vi "Flow_2_Buffer_Dbl_VIG.vi"(7 "Operation":enum16{"get data", "set data", "initialize"}(ring)=enum."set data", 8 "error in":errorcluster, 11 "Freq":dbl) -> (0 "error out":errorcluster, 3 "Raw Flow Freq":dbl)   [LabVIEW 2018]
uses:
  <vilib>/Analysis/baseanly.llb/Mean (DBL).vi
  <vilib>/measure/macond.llb/FIR Filter for 1 Chan.vi
  Common/Globals/Flow Global.vi
  <vilib>/gmath/NI_Gmath.lvlib
  <vilib>/measure/NI_MAPro.lvlib
  <vilib>/Analysis/NI_AALBase.lvlib
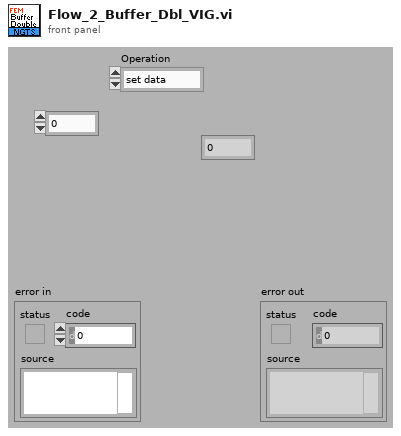
[diagram p1: front panel]
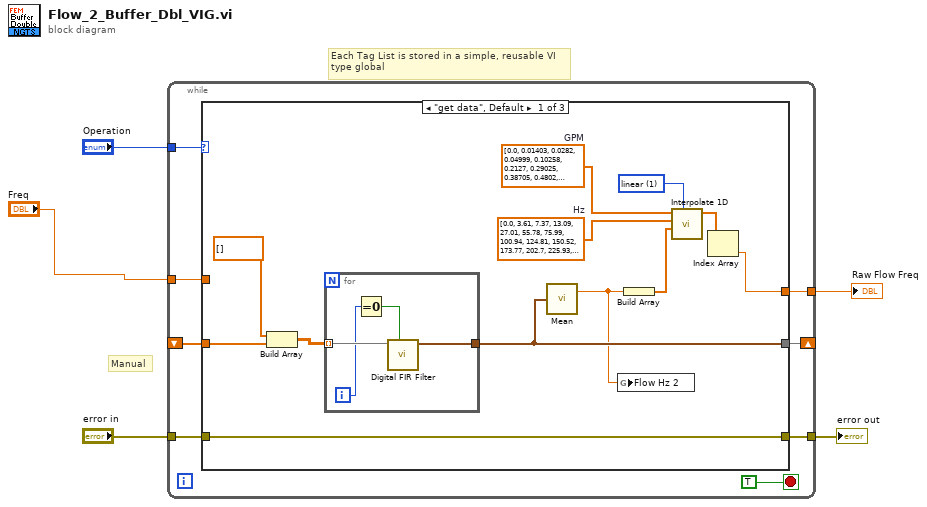
[diagram p0: block diagram]
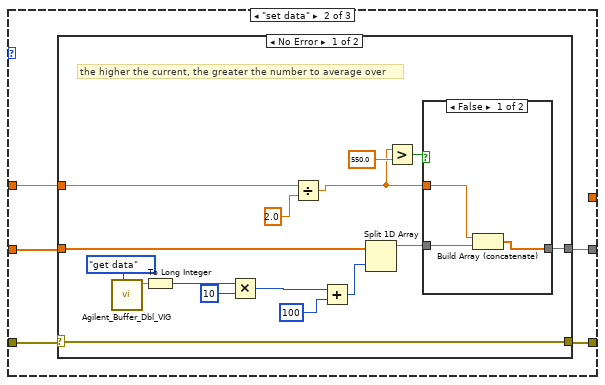
[diagram p2: hidden frame]
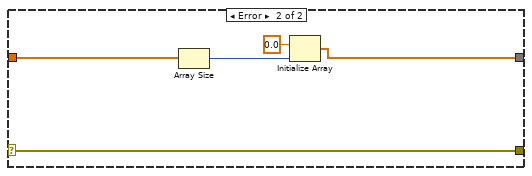
[diagram p4: hidden frame]
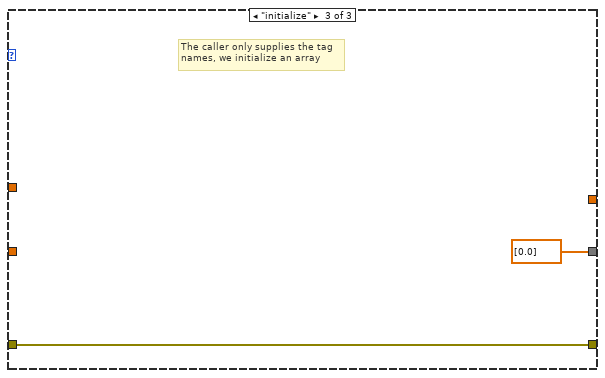
[diagram p5: hidden frame]
diagram:
  # "Manual"
  # "Each Tag List is stored in a simple, reusable VI\ntype global"
  n1 = while {
    tunnel: "Operation" -> [w13]
    tunnel: "Freq" -> [w11]
    tunnel: "error in" -> [w10]
    tunnel: [w9] -> w3
    shift-right: [w8] -> _
    shift-left: _ -> [w7]
    tunnel: [w6] -> w2
    stop <- TRUE stop-if-true
    n2 = case shown="\"get data\", Default" w13 {
      tunnel: w11 -> [_ w32 _]
      tunnel: w10 -> [w25 w31 w61]
      tunnel: [w25 w30 w61] -> w9
      tunnel: [w15 w34 dbl[] [0.0] ("Array")] -> w8
      tunnel: w7 -> [w18 w33 _]
      tunnel: [w21 _ _] -> w6
      frame "get data", Default {
        w19 = dbl[] [0.0, 0.01403, 0.0282, 0.04999, 0.10258, 0.2127, 0.29025, 0.38705, 0.4802, 0.58116, 0.67343, 0.78891, 0.88241, 0.99458, 1.0892, 1.18752, 1.40024, 1.49696, 1.61641, 1.82395, 2.03827]  # GPM
        w20 = dbl[] [0.0, 3.61, 7.37, 13.09, 27.01, 55.78, 75.99, 100.94, 124.81, 150.52, 173.77, 202.7, 225.93, 253.45, 276.83, 301.27, 352.82, 375.82, 403.94, 453.6, 503.78]  # Hz
        w24 = 1 items=["nearest", "linear", "spline", "cubic Hermite", "Lagrange"] ("method")
        n3 = Build Array(dbl[] [], w18) -> (w17:dbl[][])
        n4 = for {
          tunnel: w17 -> [w28] mode=indexing
          tunnel: [w29] -> w15
          i -> [w26]
          n5 = Equal To 0?(x=w26) -> (x = 0?=w27:bool)
          n6 = call-poly <vilib>:"Digital FIR Filter.vi"("reset filter"=w27, "signal in"=w28) -> ("signal out"=w29:waveform(dbl))  [unwired: 7 in, 2 out]
        }
        n7 = call-poly <vilib>:"Mean.vi"("X"=w15) -> ("mean"=w14:dbl)  [unwired: 1 out]
        n8 = global write "Flow Global.vi" "Flow Hz 2"(w14) -> ()
        n9 = Build Array(w14) -> (w22:dbl[])
        n10 = call <vilib>:"Interpolate 1D.vi"("method"=w24, "xi"=w22, "X"=w20, "Y"=w19) -> ("yi"=w23:dbl[])  [unwired: 5 in, 2 out]
        n11 = Index Array(array=w23) -> (element=w21:dbl)  [unwired: 1 in]
      }
      frame "set data" {
        n12 = case shown="No Error" w31 {
          selector: w31 -> [w45 w59]
          tunnel: [w50 w55] -> w34
          tunnel: w33 -> [w49 w58]
          tunnel: w32 -> [w43 _]
          tunnel: [w45 w59] -> w30
          frame No Error {
            # "the higher the current, the greater the number to average over"
            n13 = call "Agilent_Buffer_Dbl_VIG.vi"("Operation"=enum16{"get data", "set data", "initialize"}."get data") -> ("Numeric"=w38:dbl)  [unwired: 9 in, 1 out]
            n14 = To Long Integer(number=w38) -> (32bit integer=w37:i32)
            n15 = Multiply(x=w37, y=10) -> (x*y=w36:i32)
            n16 = Divide(x=w43, y=2.0 ("x")) -> (x/y=w42:dbl)
            n17 = Add(x=w36, y=100 ("index")) -> (x+y=w39:i32)
            n18 = Split 1D Array(array=w49, index=w39) -> (first subarray=w48:dbl[])  [unwired: 1 out]
            n19 = Greater?(x=w42, y=550.0) -> (0:w46:bool)
            n20 = case shown="False" w46 {
              tunnel: [w53 w54] -> w50
              tunnel: w48 -> [w52 w54]
              tunnel: w42 -> [w51 _]
              frame False {
                n21 = Build Array (concatenate)(w51, w52) -> (w53:dbl[])
              }
              frame True {
              }
            }
          }
          frame Error {
            n22 = Array Size(array=w58) -> (size(s)=w57:i32)
            n23 = Initialize Array(0.0 ("element"), w57) -> (w55:dbl[])
          }
        }
      }
      frame "initialize" {
        # "The caller only supplies the tag\nnames, we initialize an array"
      }
    }
  }
  "error out" <- w3
  "Raw Flow Freq" <- w2
